vi "testExtractElementBasicType.vi"(8 "error in (no error)":errorcluster) -> (0 "error out":errorcluster)   [LabVIEW 2018]
uses:
  SALTypeGenerator/Topic/Topic.lvclass
  SALTypeGenerator/Topic/Topic.lvclass/Topic.ctl
  <vilib>/addons/_JKI Toolkits/Caraya/classes/Assert/Assert Equal Value_Variant.vi
  <vilib>/addons/_JKI Toolkits/Caraya/classes/Test/Test.lvclass
  <vilib>/addons/_JKI Toolkits/Caraya/classes/Assert/Assert.lvclass
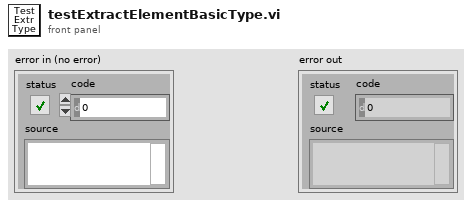
[diagram p1: front panel]
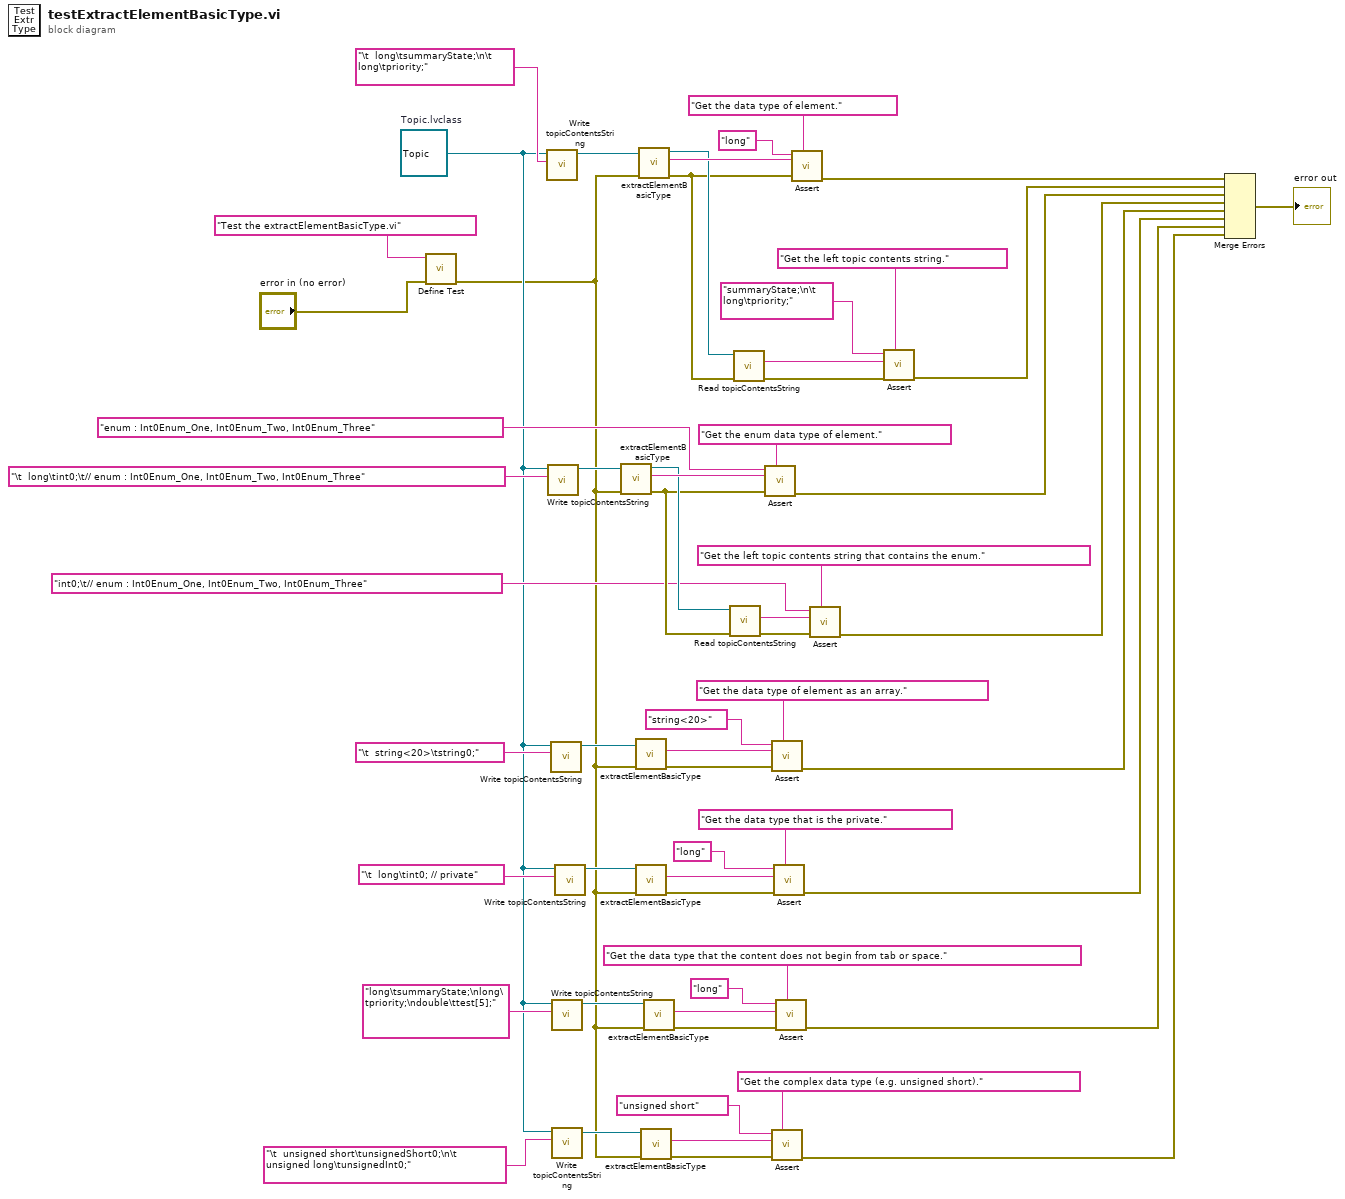
[diagram p0: block diagram]
diagram:
  w9 = refnum<class "Topic.lvclass"> refnum  # Topic.lvclass
  n1 = call <vilib>:"Define Test.vi"("error in (no error)"="error in (no error)", "Label (VI Title)"="Test the extractElementBasicType.vi") -> ("error out"=w6:errorcluster)  [unwired: 9 in]
  n2 = call "Write topicContentsString.vi"("topicContentsString"="\t  long\tsummaryState;\n\t  long\tpriority;", "Topic in"=w9) -> ("Topic out"=w56:refnum<class "Topic.lvclass">)  [unwired: 9 in]
  n3 = call "Write topicContentsString.vi"("topicContentsString"="\t  long\tint0;\t// enum : Int0Enum_One, Int0Enum_Two, Int0Enum_Three", "Topic in"=w9) -> ("Topic out"=w42:refnum<class "Topic.lvclass">)  [unwired: 9 in]
  n4 = call "Write topicContentsString.vi"("topicContentsString"="\t  string<20>\tstring0;", "Topic in"=w9) -> ("Topic out"=w36:refnum<class "Topic.lvclass">)  [unwired: 9 in]
  n5 = call "Write topicContentsString.vi"("topicContentsString"="long\tsummaryState;\nlong\tpriority;\ndouble\ttest[5];", "Topic in"=w9) -> ("Topic out"=w15:refnum<class "Topic.lvclass">)  [unwired: 9 in]
  n6 = call "Write topicContentsString.vi"("topicContentsString"="\t  unsigned short\tunsignedShort0;\n\t  unsigned long\tunsignedInt0;", "Topic in"=w9) -> ("Topic out"=w7:refnum<class "Topic.lvclass">)  [unwired: 9 in]
  n7 = call "Write topicContentsString.vi"("topicContentsString"="\t  long\tint0; // private", "Topic in"=w9) -> ("Topic out"=w22:refnum<class "Topic.lvclass">)  [unwired: 9 in]
  n8 = call "extractElementBasicType.vi"("error in (no error)"=w6, "Topic in"=w42) -> ("error out"=w30:errorcluster, "elementBasicType"=w41:string, "Topic out"=w31:refnum<class "Topic.lvclass">)  [unwired: 7 in]
  n9 = call "extractElementBasicType.vi"("error in (no error)"=w6, "Topic in"=w36) -> ("error out"=w35:errorcluster, "elementBasicType"=w34:string)  [unwired: 7 in, 1 out]
  n10 = call "extractElementBasicType.vi"("error in (no error)"=w6, "Topic in"=w22) -> ("error out"=w21:errorcluster, "elementBasicType"=w20:string)  [unwired: 7 in, 1 out]
  n11 = call "extractElementBasicType.vi"("error in (no error)"=w6, "Topic in"=w56) -> ("error out"=w51:errorcluster, "elementBasicType"=w55:string, "Topic out"=w52:refnum<class "Topic.lvclass">)  [unwired: 7 in]
  n12 = call "extractElementBasicType.vi"("error in (no error)"=w6, "Topic in"=w7) -> ("error out"=w5:errorcluster, "elementBasicType"=w4:string)  [unwired: 7 in, 1 out]
  n13 = call "extractElementBasicType.vi"("error in (no error)"=w6, "Topic in"=w15) -> ("error out"=w14:errorcluster, "elementBasicType"=w13:string)  [unwired: 7 in, 1 out]
  n14 = call "Read topicContentsString.vi"("error in (no error)"=w30, "Topic in"=w31) -> ("error out"=w29:errorcluster, "topicContentsString"=w28:string)  [unwired: 7 in, 1 out]
  n15 = call "Read topicContentsString.vi"("error in (no error)"=w51, "Topic in"=w52) -> ("error out"=w50:errorcluster, "topicContentsString"=w49:string)  [unwired: 7 in, 1 out]
  n16 = call-poly <vilib>:"Assert.vi"("Label"="Get the enum data type of element.", "error in (no error)"=w30, "Y"=w41, "X"="enum : Int0Enum_One, Int0Enum_Two, Int0Enum_Three") -> ("error out"=w39:errorcluster)  [unwired: 7 in]
  n17 = call-poly <vilib>:"Assert.vi"("Label"="Get the data type of element as an array.", "error in (no error)"=w35, "Y"=w34, "X"="string<20>") -> ("error out"=w24:errorcluster)  [unwired: 7 in]
  n18 = call-poly <vilib>:"Assert.vi"("Label"="Get the complex data type (e.g. unsigned short).", "error in (no error)"=w5, "Y"=w4, "X"="unsigned short") -> ("error out"=w1:errorcluster)  [unwired: 7 in]
  n19 = call-poly <vilib>:"Assert.vi"("Label"="Get the data type that is the private.", "error in (no error)"=w21, "Y"=w20, "X"="long") -> ("error out"=w17:errorcluster)  [unwired: 7 in]
  n20 = call-poly <vilib>:"Assert.vi"("Label"="Get the data type that the content does not begin from tab or space.", "error in (no error)"=w14, "Y"=w13, "X"="long") -> ("error out"=w10:errorcluster)  [unwired: 7 in]
  n21 = call-poly <vilib>:"Assert.vi"("Label"="Get the data type of element.", "error in (no error)"=w51, "Y"=w55, "X"="long") -> ("error out"=w46:errorcluster)  [unwired: 7 in]
  n22 = call-poly <vilib>:"Assert.vi"("Label"="Get the left topic contents string that contains the enum.", "error in (no error)"=w29, "Y"=w28, "X"="int0;\t// enum : Int0Enum_One, Int0Enum_Two, Int0Enum_Three") -> ("error out"=w25:errorcluster)  [unwired: 7 in]
  n23 = call-poly <vilib>:"Assert.vi"("Label"="Get the left topic contents string.", "error in (no error)"=w50, "Y"=w49, "X"="summaryState;\n\t  long\tpriority;") -> ("error out"=w45:errorcluster)  [unwired: 7 in]
  n24 = Merge Errors(w46, w45, w39, w25, w24, w17, w10, w1) -> (→"error out":errorcluster)
